vi "4-1 somma-differenza - vettorelink.vi"(2 "vet b":dbl[](array[numeric]) format="%.2f", 3 "const":dbl format="%.2f", 4 "vet a":dbl[](array[numeric]) format="%.2f") -> (0 "vet link":dbl[](array[numeric]) format="%.2f", 1 "vet som-diff":dbl[](array[numeric]) format="%.2f")   [LabVIEW 2012]
doc: "M. Ferrari Vet Func Ex"
panel:
  # "1° fase\nPER OGNI COMPONENTE DEI VETTORI di INGRESSO \nviene calcolata LA SOMMA se vet a (I)<vet b (I),\naltrimenti LA DIFFERENZA delle due componenti;\nIl risultato sarà presente in vet som-diff."
  # "2° fase\nL'ultima componente di vet som-diff dovrà essere\nsostituita con il valore di const; si vuol creare un nuovo\nvettore, vet link, come risultato della concatenazione\n di vet a, di const(scalare), e di vet som-diff\n(dopo la modifica iniziale sull'ultima componente)."
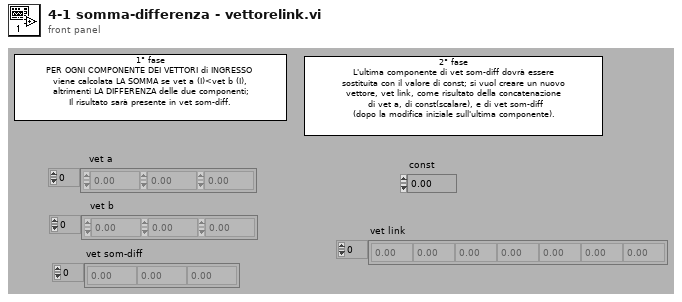
[diagram p1: front panel]
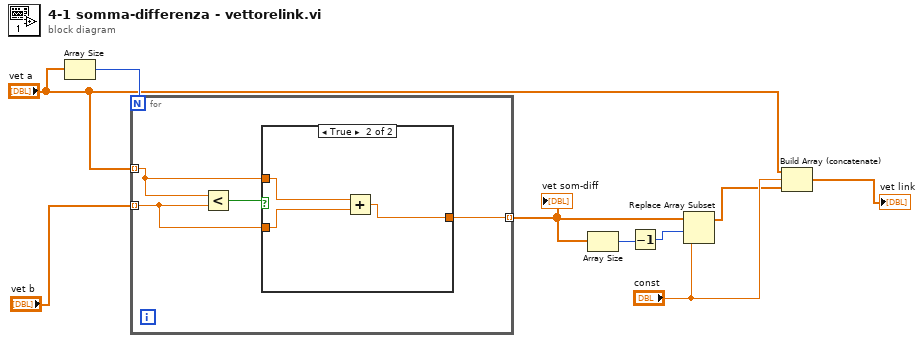
[diagram p0: block diagram]
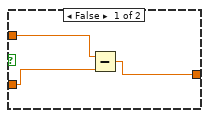
[diagram p2: hidden frame]
diagram:
  n1 = Array Size(array="vet a") -> (size(s)=w6:i32)
  n2 = for {
    N: w6 -> [_]
    tunnel: [w12] -> w3 mode=indexing
    tunnel: "vet a" -> [w11] mode=indexing
    tunnel: "vet b" -> [w10] mode=indexing
    n3 = Less?(x=w11, y=w10) -> (x < y?=w13:bool)
    n4 = case shown="True" w13 {
      tunnel: [w16 w19] -> w12
      tunnel: w11 -> [w15 w18]
      tunnel: w10 -> [w14 w17]
      frame False {
        n5 = Subtract(x=w15, y=w14) -> (x-y=w16:dbl)
      }
      frame True {
        n6 = Add(x=w18, y=w17) -> (x+y=w19:dbl)
      }
    }
  }
  "vet som-diff" <- w3
  n7 = Array Size(array=w3) -> (size(s)=w2:i32)
  n8 = Decrement(x=w2) -> (x-1=w1:i32)
  n9 = Replace Array Subset(array=w3, new element="const", index=w1) -> (w8:dbl[])
  n10 = Build Array (concatenate)("vet a", "const", w8) -> (→"vet link":dbl[])
